vi "Single DM Control.vi"() -> ()   [LabVIEW 2016]
uses:
  Controls/Pixel Scan Parameters.ctl
  Controls/MirrorModes.ctl
  Hardware Configuration/Hardware Configuration Controls/Standard Action.ctl
  <vilib>/Analysis/baseanly.llb/Mean (DBL).vi
  <vilib>/Utility/file.llb/Write Delimited Spreadsheet (DBL).vi
  <vilib>/Utility/file.llb/Read Delimited Spreadsheet (DBL).vi
  <vilib>/Analysis/NI_AALBase.lvlib
panel:
  in  "Load Control Matrix":bool
  in  "Bias Level":dbl format="%#_13g"
  in  "Load Flat":bool
  in  "Apply Zero":bool
  in  "Load V Map":bool
  in  "Save V Map":bool
  in  "Apply Flat":bool
  in  "Center Bias":bool
  in  "Exit":bool
  in  "Mirror Tab":enum32{"Mirror Modes", "Scan Pixels", "Poke"}(tab)
  in  "Clear Modes":bool
  in  "Mirror Modes":T1
  in  "Load Modes":bool
  in  "Save Modes":bool
  in  "Scan Modes":bool
  in  "Pixel Scan Save Path":path
  in  "Save Data":bool
  in  "Pixel Scan Parameters":T2={"Scan Start Pixel"=1, "Scan End Pixel"=1, "Pixel Start Value (-1 to 1)"=-0.5, "Pixel End Value (-1 to 1)"=0.5, "Number of Steps"=0.1}
  in  "Start Pixel Scan":bool
  in  "Poke Amount":dbl=1.0
  in  "Pixel No.":i32=1
  in  "Poke":bool
  in  "Poke Unit":T3(radio)
  out "Pixel Map (-1 to 1)":dbl[][](graph)
  # "Mode"
  # "Amount (nm)"
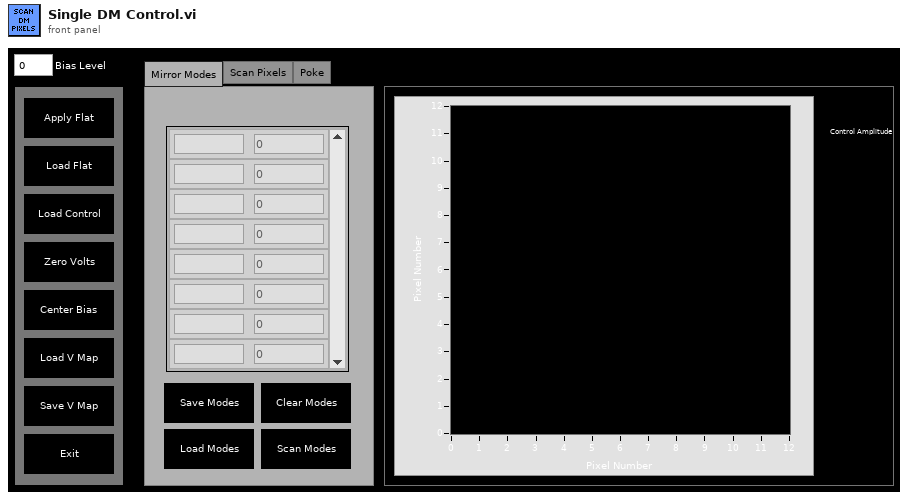
[diagram p1: front panel]
types:
  T1 = typedef "MirrorModes.ctl" = cluster{"Mode":string, "Amplitude":dbl}[]
  T2 = typedef "Pixel Scan Parameters.ctl" = cluster{"Scan Start Pixel":i32, "Scan End Pixel":i32, "Pixel Start Value (-1 to 1)":dbl, "Pixel End Value (-1 to 1)":dbl, "Number of Steps":dbl}
  T3 = enum32{"Voltage (V)", "Control Parameter [-1, 1]", "Approx. Distance (nm)"}
  T4 = typedef "Standard Action.ctl" = enum16{"Read", "Write"}
  T5 = enum16{"Start Scan", "Reset Counter", "Write DM", "Get Image", "Update Count", "Exit"}
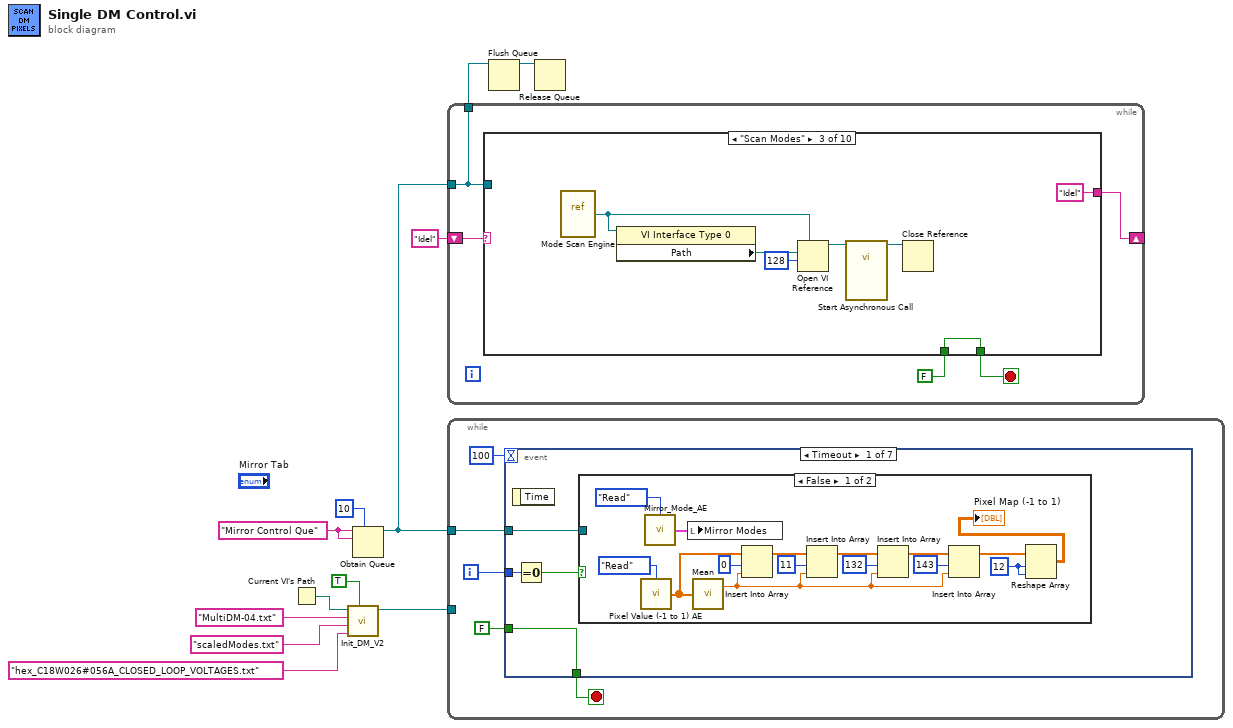
[diagram p0: block diagram]
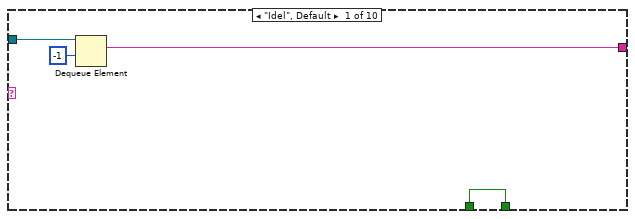
[diagram p2: hidden frame]
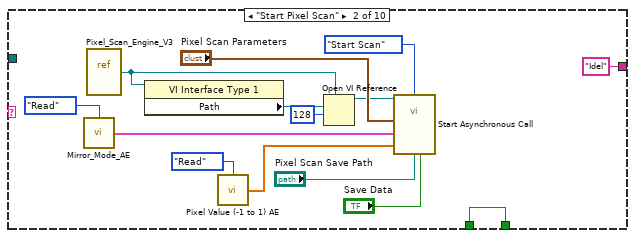
[diagram p3: hidden frame]
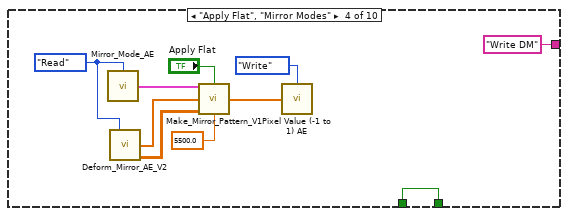
[diagram p4: hidden frame]
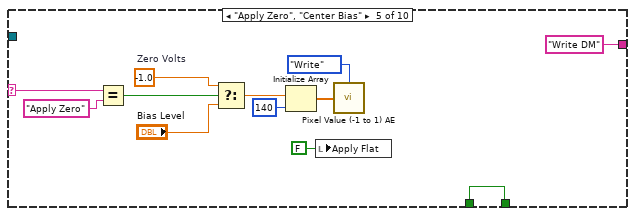
[diagram p5: hidden frame]
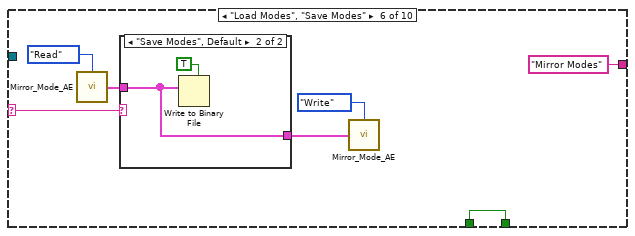
[diagram p6: hidden frame]
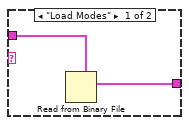
[diagram p7: hidden frame]
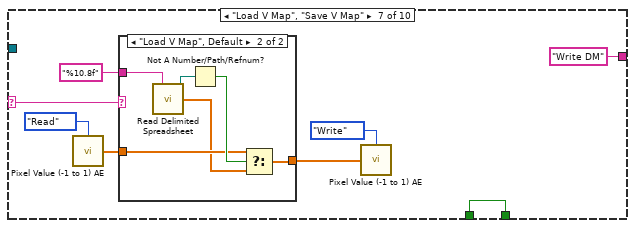
[diagram p8: hidden frame]
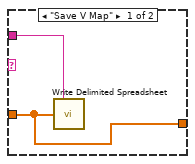
[diagram p9: hidden frame]
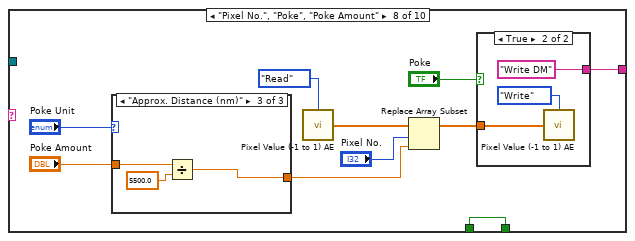
[diagram p10: hidden frame]
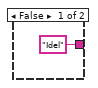
[diagram p11: hidden frame]
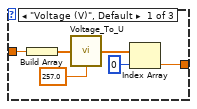
[diagram p12: hidden frame]
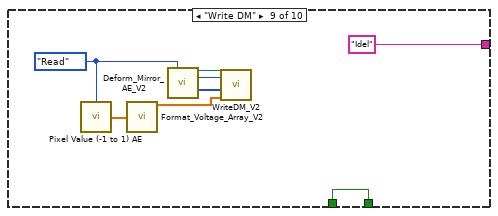
[diagram p14: hidden frame]
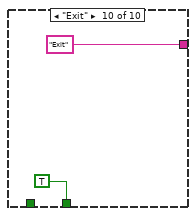
[diagram p15: hidden frame]
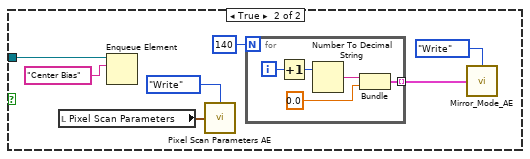
[diagram p16: hidden frame]
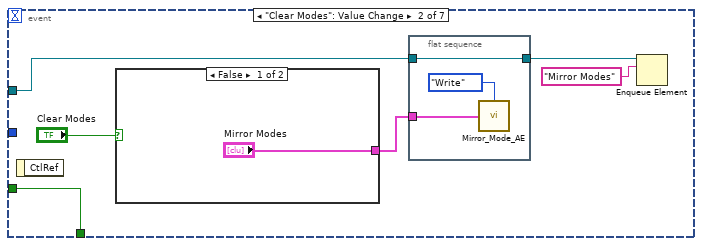
[diagram p17: hidden frame]
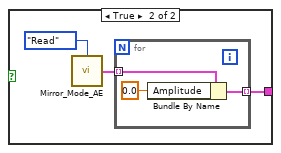
[diagram p18: hidden frame]
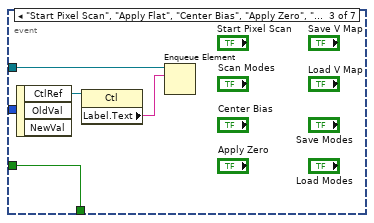
[diagram p19: hidden frame]
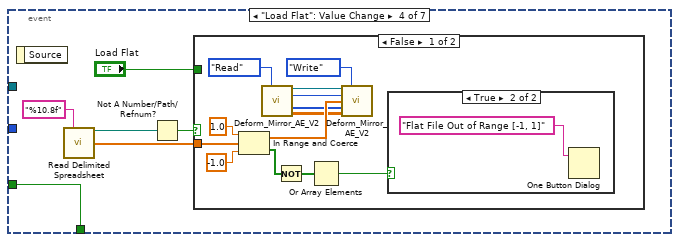
[diagram p20: hidden frame]
diagram:
  w12 = "Mirror Control Que" ("name (unnamed)")
  n1 = Current VI's Path() -> (path=w4:path)
  n2 = call "Init_DM_V2.vi"("BM Flat"=TRUE, "BM Flat File"="hex_C18W026#056A_CLOSED_LOOP_VOLTAGES.txt" ("name or relative path"), "Mirror Modes File"="scaledModes.txt" ("name or relative path"), "DM Mapping File"="MultiDM-04.txt" ("name or relative path"), "Base File Path"=w4) -> ("reference out"=w10:refnum<k7>)  [unwired: 6 in]
  n3 = Obtain Queue(max queue size (-1, unlimited)=10, name (unnamed)=w12, element data type=w12) -> (queue out=w6:refnum<queue>)  [unwired: 2 in, 2 out]
  n4 = while {
    tunnel: w6 -> [w13]
    shift-right: [w17] -> _
    shift-left: "Idel" ("name (unnamed)") -> [w16]
    tunnel: [w13] -> w9
    stop <- w15 stop-if-true
    n5 = case shown="\"Scan Modes\"" w16 {
      selector: w16 -> [_ _ _ _ w59 w67 w82 _ _ _]
      tunnel: w13 -> [w21 _ _ _ _ _ _ _ _ _]
      tunnel: [w19 "Idel" ("name (unnamed)") "Idel" ("name (unnamed)") "Write DM" ("name (unnamed)") "Write DM" ("name (unnamed)") "Mirror Modes" ("name (unnamed)") "Write DM" ("name (unnamed)") w93 "Idel" ("name (unnamed)") "Exit" ("name (unnamed)")] -> w17
      tunnel: [w18 w35 w42 w51 w64 w71 w83 w101 w123 TRUE] -> w15
      tunnel: FALSE -> [w18 w35 w42 w51 w64 w71 w83 w101 w123 _]
      frame "Idel", Default {
        n6 = Dequeue Element(queue=w21, timeout in ms (-1)=-1) -> (element=w19:string)  [unwired: 1 in, 3 out]
      }
      frame "Start Pixel Scan" {
        n7 = call "Mirror_Mode_AE.vi"("Action"=Standard_Action."Read") -> ("Mirror Modes Out"=w22:T1)  [unwired: 14 in]
        n8 = vi-ref "Pixel_Scan_Engine_V3.vi"() -> (w26:refnum<vi>)
        n9 = property class="VI Interface Type 1"(reference=w26) -> ("Path"=w24:path)  [unwired: 1 in, 2 out]
        n10 = call "Pixel Value (-1 to 1) AE.vi"("Action"=Standard_Action."Read") -> ("Pixel Value (-1 to 1) Out"=w33:dbl[])  [unwired: 14 in]
        n11 = Open VI Reference(type specifier VI Refnum (for type only)=w26, vi path=w24, options=128) -> (vi reference=w27:refnum<vi>)  [unwired: 3 in, 1 out]
        n12 = call-by-ref "Start Asynchronous Call"(reference=w27, "Pixel Scan Parameters In"="Pixel Scan Parameters", "Action"=T5."Start Scan", "Initial Mirror Modes"=w22, "Initial Pixel Values (-1 to 1)"=w33, "Base Save Path"="Pixel Scan Save Path", "Save Data"="Save Data") -> ()  [unwired: 11 in, 2 out]
      }
      frame "Scan Modes" {
        n13 = vi-ref "Mode Scan Engine.vi"() -> (w36:refnum<vi>)
        n14 = property class="VI Interface Type 0"(reference=w36) -> ("Path"=w37:path)  [unwired: 1 in, 2 out]
        n15 = Open VI Reference(type specifier VI Refnum (for type only)=w36, vi path=w37, options=128) -> (vi reference=w39:refnum<vi>)  [unwired: 3 in, 1 out]
        n16 = call-by-ref "Start Asynchronous Call"(reference=w39) -> (reference out=w40:refnum<vi>)  [unwired: 17 in, 1 out]
        n17 = Close Reference(reference=w40) -> ()  [unwired: 1 in, 1 out]
      }
      frame "Apply Flat", "Mirror Modes" {
        w45 = Standard_Action."Read" ("Action")
        n18 = call "Mirror_Mode_AE.vi"("Action"=w45) -> ("Mirror Modes Out"=w48:T1)  [unwired: 14 in]
        n19 = call "Deform_Mirror_AE_V2.vi"("Action"=w45) -> ("Flat Files Out"=w49:dbl[], "Mode Matrix Out"=w50:dbl[][])  [unwired: 10 in, 3 out]
        n20 = call "Make_Mirror_Pattern_V1.vi"("Mirror Modes In"=w48, "Flat On?"="Apply Flat", "Flat File In"=w49, "Mirror Modes Array"=w50, "Amplitude Scale Factor"=5500.0) -> ("Pixel Value U (-1 to 1)"=w47:dbl[])  [unwired: 10 in]
        n21 = call "Pixel Value (-1 to 1) AE.vi"("Action"=Standard_Action."Write", "Pixel Value (-1 to 1)"=w47) -> ()  [unwired: 13 in, 1 out]
      }
      frame "Apply Zero", "Center Bias" {
        w55 = -1.0  # Zero Volts
        n22 = Equal?(x=w59, y="Apply Zero") -> (x = y?=w58:bool)
        n23 = Select(t=w55, s=w58, f="Bias Level") -> (s? t:f=w56:dbl)
        n24 = Initialize Array(w56, 140 ("dimension size")) -> (w62:dbl[])
        n25 = local write "Apply Flat"(FALSE ("Apply Flat")) -> ()
        n26 = call "Pixel Value (-1 to 1) AE.vi"("Action"=Standard_Action."Write", "Pixel Value (-1 to 1)"=w62) -> ()  [unwired: 13 in, 1 out]
      }
      frame "Load Modes", "Save Modes" {
        n27 = call "Mirror_Mode_AE.vi"("Action"=Standard_Action."Read") -> ("Mirror Modes Out"=w66:T1)  [unwired: 14 in]
        n28 = case shown="\"Save Modes\", Default" w67 {
          tunnel: w66 -> [w73 w74]
          tunnel: [w72 w74] -> w65
          frame "Load Modes" {
            n29 = Read from Binary File(5:w73) -> (2:w72:T1)  [unwired: 5 in, 3 out]
          }
          frame "Save Modes", Default {
            n30 = Write to Binary File(data=w74, 5:TRUE ("prepend array or string size? (T)")) -> ()  [unwired: 4 in, 3 out]
          }
        }
        n31 = call "Mirror_Mode_AE.vi"("Action"=Standard_Action."Write", "Mirror Modes In"=w65) -> ()  [unwired: 13 in, 1 out]
      }
      frame "Load V Map", "Save V Map" {
        n32 = call "Pixel Value (-1 to 1) AE.vi"("Action"=Standard_Action."Read") -> ("Pixel Value (-1 to 1) Out"=w80:dbl[])  [unwired: 14 in]
        n33 = case shown="\"Load V Map\", Default" w82 {
          tunnel: w80 -> [w84 w88]
          tunnel: "%10.8f" -> [w85 w91]
          tunnel: [w84 w86] -> w76
          frame "Save V Map" {
            n34 = call-poly <vilib>:"Write Delimited Spreadsheet.vi"("format (%.3f)"=w85, "1D data"=w84) -> ()  [unwired: 12 in, 2 out]
          }
          frame "Load V Map", Default {
            n35 = call-poly <vilib>:"Read Delimited Spreadsheet.vi"("format (%.3f)"=w91) -> ("new file path (Not A Path if cancelled)"=w90:path, "first row"=w87:dbl[])  [unwired: 9 in, 4 out]
            n36 = Not A Number/Path/Refnum?(number/path/refnum=w90) -> (NaN/Path/Refnum?=w89:bool)
            n37 = Select(t=w88, s=w89, f=w87) -> (s? t:f=w86:dbl[])
          }
        }
        n38 = call "Pixel Value (-1 to 1) AE.vi"("Action"=Standard_Action."Write", "Pixel Value (-1 to 1)"=w76) -> ()  [unwired: 13 in, 1 out]
      }
      frame "Pixel No.", "Poke", "Poke Amount" {
        n39 = case shown="\"Approx. Distance (nm)\"" "Poke Unit" {
          tunnel: "Poke Amount" -> [w110 w112 w115]
          tunnel: [w106 w112 w113] -> w99
          frame "Voltage (V)", Default {
            n40 = Build Array(w110) -> (w109:dbl[])
            n41 = call "Voltage_To_U.vi"("Voltages In (Volts)"=w109, "Mirror Max Voltage (Volts)"=257.0) -> ("Pixel Value (-1 to 1)"=w108:dbl[])  [unwired: 13 in]
            n42 = Index Array(array=w108, index=0) -> (element=w106:dbl)
          }
          frame "Control Parameter [-1, 1]" {
          }
          frame "Approx. Distance (nm)" {
            n43 = Divide(x=w115, y=5500.0) -> (x/y=w113:dbl)
          }
        }
        n44 = call "Pixel Value (-1 to 1) AE.vi"("Action"=Standard_Action."Read") -> ("Pixel Value (-1 to 1) Out"=w100:dbl[])  [unwired: 14 in]
        n45 = Replace Array Subset(array=w100, new element=w99, index="Pixel No.") -> (w94:dbl[])
        n46 = case shown="True" "Poke" {
          tunnel: w94 -> [_ w104]
          tunnel: ["Idel" ("name (unnamed)") "Write DM" ("name (unnamed)")] -> w93
          frame False {
          }
          frame True {
            n47 = call "Pixel Value (-1 to 1) AE.vi"("Action"=Standard_Action."Write", "Pixel Value (-1 to 1)"=w104) -> ()  [unwired: 13 in, 1 out]
          }
        }
      }
      frame "Write DM" {
        w121 = Standard_Action."Read" ("Action")
        n48 = call "Pixel Value (-1 to 1) AE.vi"("Action"=w121) -> ("Pixel Value (-1 to 1) Out"=w120:dbl[])  [unwired: 14 in]
        n49 = call "Format_Voltage_Array_V2.vi"("Pixel Level (-1 to 1)"=w120) -> ("Voltage Array (Volts)"=w116:dbl[])  [unwired: 13 in, 1 out]
        n50 = call "Deform_Mirror_AE_V2.vi"("Action"=w121) -> ("Refnum Out"=w119:refnum<k7>, "IDs Out"=w118:i32, "Multi Map Data Out"=w117:i32[])  [unwired: 10 in, 2 out]
        n51 = call "WriteDM_V2.vi"("reference in"=w119, "nDevId"=w118, "MultiDM  Mapping"=w117, "Voltage Array in"=w116) -> ()  [unwired: 2 in, 2 out]
      }
      frame "Exit" {
      }
    }
  }
  n52 = while {
    tunnel: w6 -> [w126]
    tunnel: w10 -> [_]
    i -> [w127]
    stop <- w130 stop-if-true
    n53 = event shown="[0] Timeout" {
      selector: _ -> [_ _ _ _ _ _ _]
      dyn-events: _ -> [_ _ _ _ _ _ _]
      timeout: 100 -> [_ _ _ _ _ _ _]
      tunnel: [w134 w167 w181 w187 w206 w220 w242] -> w130
      tunnel: FALSE -> [w134 w167 w181 w187 w206 w220 _]
      tunnel: w127 -> [w133 _ _ _ _ _ _]
      tunnel: w126 -> [w131 w166 w180 _ _ _ w240]
      event Timeout {
        n54 = event-data() -> ()  [unwired: 1 in, 1 out]
        n55 = Equal To 0?(x=w133) -> (x = 0?=w132:bool)
        n56 = case shown="False" w132 {
          tunnel: w131 -> [_ w156]
          frame False {
            w148 = 12 ("dimension size")
            n57 = call "Pixel Value (-1 to 1) AE.vi"("Action"=Standard_Action."Read") -> ("Pixel Value (-1 to 1) Out"=w149:dbl[])  [unwired: 14 in]
            n58 = call "Mirror_Mode_AE.vi"("Action"=Standard_Action."Read") -> ("Mirror Modes Out"=w136:T1)  [unwired: 14 in]
            n59 = local write "Mirror Modes"(w136) -> ()
            n60 = call-poly <vilib>:"Mean.vi"("X"=w149) -> ("mean"=w146:dbl)  [unwired: 1 out]
            n61 = Insert Into Array(array=w149, index=0, new element=w146) -> (w141:dbl[])
            n62 = Insert Into Array(array=w141, index=11, new element=w146) -> (w143:dbl[])
            n63 = Insert Into Array(array=w143, index=132, new element=w146) -> (w145:dbl[])
            n64 = Insert Into Array(array=w145, index=143, new element=w146) -> (w138:dbl[])
            n65 = Reshape Array(w138, w148, w148) -> (→"Pixel Map (-1 to 1)":dbl[][])
          }
          frame True {
            n66 = local read "Pixel Scan Parameters"() -> (w153:T2)
            n67 = Enqueue Element(queue=w156, element="Center Bias") -> ()  [unwired: 2 in, 3 out]
            n68 = call "Pixel Scan Parameters AE.vi"("Action"=enum16{"Write", "Read"}."Write", "Pixel Scan Parameters"=w153) -> ()  [unwired: 13 in, 1 out]
            n69 = for {
              N: 140 -> [_]
              tunnel: [w157] -> w150 mode=indexing
              i -> [w161]
              n70 = Increment(x=w161) -> (x+1=w160:i32)
              n71 = Number To Decimal String(number=w160) -> (decimal integer string=w159:string)  [unwired: 1 in]
              n72 = Bundle(w159, 0.0) -> (w157:cluster{string, dbl})  [unwired: 1 in]
            }
            n73 = call "Mirror_Mode_AE.vi"("Action"=Standard_Action."Write", "Mirror Modes In"=w150) -> ()  [unwired: 13 in, 1 out]
          }
        }
      }
      event "Clear Modes": Value Change {
        n74 = event-data() -> ()  [unwired: 1 in, 1 out]
        n75 = case shown="False" "Clear Modes" {
          tunnel: ["Mirror Modes" w169] -> w162
          frame False {
          }
          frame True {
            n76 = call "Mirror_Mode_AE.vi"("Action"=Standard_Action."Read") -> ("Mirror Modes Out"=w171:T1)  [unwired: 14 in]
            n77 = for {
              tunnel: w171 -> [w174] mode=indexing
              tunnel: [w172] -> w169 mode=indexing
              n78 = Bundle By Name(cluster=w174, "Amplitude"=0.0) -> (w172:cluster{"Mode":string, "Amplitude":dbl})
            }
          }
        }
        n79 = flat-sequence {
          tunnel: w162 -> [w176]
          tunnel: w166 -> [w175]
          tunnel: [w175] -> w164
          frame #0 {
            n80 = call "Mirror_Mode_AE.vi"("Action"=Standard_Action."Write", "Mirror Modes In"=w176) -> ()  [unwired: 13 in, 1 out]
          }
        }
        n81 = Enqueue Element(queue=w164, element="Mirror Modes") -> ()  [unwired: 2 in, 3 out]
      }
      event "Start Pixel Scan", "Apply Flat", "Center Bias", "Apply Zero", "Save V Map", "Save Modes", "Load Modes", "Load V Map", "Scan Modes", "Poke", "Pixel No.", "Poke Amount": Value Change {
        n82 = event-data() -> ("CtlRef"=w179:refnum<vi>)  [unwired: 1 in, 2 out]
        n83 = property class="Ctl"(reference=w179) -> ("Label.Text"=w178:string)  [unwired: 1 in, 2 out]
        n84 = Enqueue Element(queue=w180, element=w178) -> ()  [unwired: 2 in, 3 out]
      }
      event "Load Flat": Value Change {
        n85 = event-data() -> ()  [unwired: 1 in, 1 out]
        n86 = call-poly <vilib>:"Read Delimited Spreadsheet.vi"("format (%.3f)"="%10.8f") -> ("new file path (Not A Path if cancelled)"=w183:path, "first row"=w182:dbl[])  [unwired: 9 in, 4 out]
        n87 = Not A Number/Path/Refnum?(number/path/refnum=w183) -> (NaN/Path/Refnum?=w186:bool)
        n88 = case shown="False" w186 {
          tunnel: w182 -> [w200 _]
          tunnel: "Load Flat" -> [_ _]
          frame False {
            n89 = In Range and Coerce(upper limit=1.0, x=w200, lower limit=-1.0) -> (coerced(x)=w193:dbl[], In Range?=w197:bool[])
            n90 = call "Deform_Mirror_AE_V2.vi"("Action"=Standard_Action."Read") -> ("Refnum Out"=w189:refnum<k7>, "IDs Out"=w190:i32, "Multi Map Data Out"=w191:i32[], "Mode Matrix Out"=w192:dbl[][])  [unwired: 10 in, 1 out]
            n91 = Not(x=w197) -> (.not. x?=w196:bool[])
            n92 = Or Array Elements(Boolean array=w196) -> (logical OR=w188:bool)
            n93 = call "Deform_Mirror_AE_V2.vi"("Refnum In"=w189, "Action"=Standard_Action."Write", "IDs In"=w190, "Flat Files In"=w193, "Multi Map Data In"=w191, "Mode Matrix"=w192) -> ()  [unwired: 5 in, 5 out]
            n94 = case shown="True" w188 {
              frame False {
              }
              frame True {
                n95 = One Button Dialog(message="Flat File Out of Range [-1, 1]") -> ()  [unwired: 1 in, 1 out]
              }
            }
          }
          frame True {
          }
        }
      }
      event "Load Control Matrix": Value Change {
        n96 = event-data() -> ()  [unwired: 1 in, 1 out]
        n97 = call-poly <vilib>:"Read Delimited Spreadsheet.vi"("format (%.3f)"="%10.8f") -> ("new file path (Not A Path if cancelled)"=w205:path, "all rows"=w202:dbl[][])  [unwired: 9 in, 4 out]
        n98 = Not A Number/Path/Refnum?(number/path/refnum=w205) -> (NaN/Path/Refnum?=w203:bool)
        n99 = case shown="True" w203 {
          tunnel: w202 -> [_ w207]
          frame False {
          }
          frame True {
            n100 = call "Deform_Mirror_AE_V2.vi"("Action"=Standard_Action."Read") -> ("Refnum Out"=w210:refnum<k7>, "IDs Out"=w211:i32, "Flat Files Out"=w212:dbl[], "Multi Map Data Out"=w213:i32[])  [unwired: 10 in, 1 out]
            n101 = call "Deform_Mirror_AE_V2.vi"("Refnum In"=w210, "Action"=Standard_Action."Write", "IDs In"=w211, "Flat Files In"=w212, "Multi Map Data In"=w213, "Mode Matrix"=w207) -> ()  [unwired: 5 in, 5 out]
          }
        }
      }
      event "Poke Unit": Value Change {
        n102 = event-data() -> ("NewVal"=w218:T3)  [unwired: 1 in]
        n103 = local read "Pixel No."() -> (w214:i32)
        n104 = call "Pixel Value (-1 to 1) AE.vi"("Action"=Standard_Action."Read") -> ("Pixel Value (-1 to 1) Out"=w217:dbl[])  [unwired: 14 in]
        n105 = Index Array(array=w217, index=w214) -> (element=w216:dbl)
        n106 = case shown="\"Voltage (V)\", Default" w218 {
          tunnel: w216 -> [w225 w226 w229]
          tunnel: [w223 w226 w227] -> w215
          frame "Voltage (V)", Default {
            n107 = Build Array(w225) -> (w222:dbl[])
            n108 = call "Format_Voltage_Array_V2.vi"("Pixel Level (-1 to 1)"=w222) -> ("Voltage Array (Volts)"=w221:dbl[])  [unwired: 13 in, 1 out]
            n109 = Index Array(array=w221, index=0) -> (element=w223:dbl)
          }
          frame "Control Parameter [-1, 1]" {
          }
          frame "Approx. Distance (nm)" {
            n110 = Divide(x=w229, y=5500.0) -> (x/y=w227:dbl)
          }
        }
        n111 = local write "Poke Amount"(w215) -> ()
      }
      event "Exit": Value Change {
        n112 = event-data() -> ("NewVal"=w242:bool)  [unwired: 1 in]
        n113 = Enqueue Element(queue=w240, element="Apply Zero") -> (queue out=w239:refnum<queue>)  [unwired: 2 in, 2 out]
        n114 = Enqueue Element(queue=w239, element="Exit") -> (error out=w231:errorcluster)  [unwired: 2 in, 2 out]
        n115 = call "Deform_Mirror_AE_V2.vi"("Action"=Standard_Action."Read") -> ("Refnum Out"=w234:refnum<k7>, "IDs Out"=w235:i32)  [unwired: 10 in, 3 out]
        n116 = Build Array(w235) -> (w236:i32[])
        n117 = call "ConfigDM.vi"("High Voltage"=FALSE, "error in (no error)"=w231, "Dev IDs"=w236, "Automation Refnum in"=w234) -> ("error out"=w230:errorcluster, "Automation Refnum out"=w233:refnum<k7>)  [unwired: 6 in]
        n118 = Close Reference(reference=w233, error in (no error)=w230) -> ()  [unwired: 1 out]
      }
    }
  }
  n119 = Flush Queue(queue=w9) -> (queue out=w8:refnum<queue>)  [unwired: 1 in, 2 out]
  n120 = Release Queue(queue=w8) -> ()  [unwired: 2 in, 3 out]
